vi "Error Manager Main.vi"(8 "error in (no error)":errorcluster) -> ()   [LabVIEW 2019]
uses:
  Stop Button/SubVI/Get Stop Button Status.vi
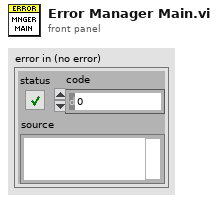
[diagram p1: front panel]
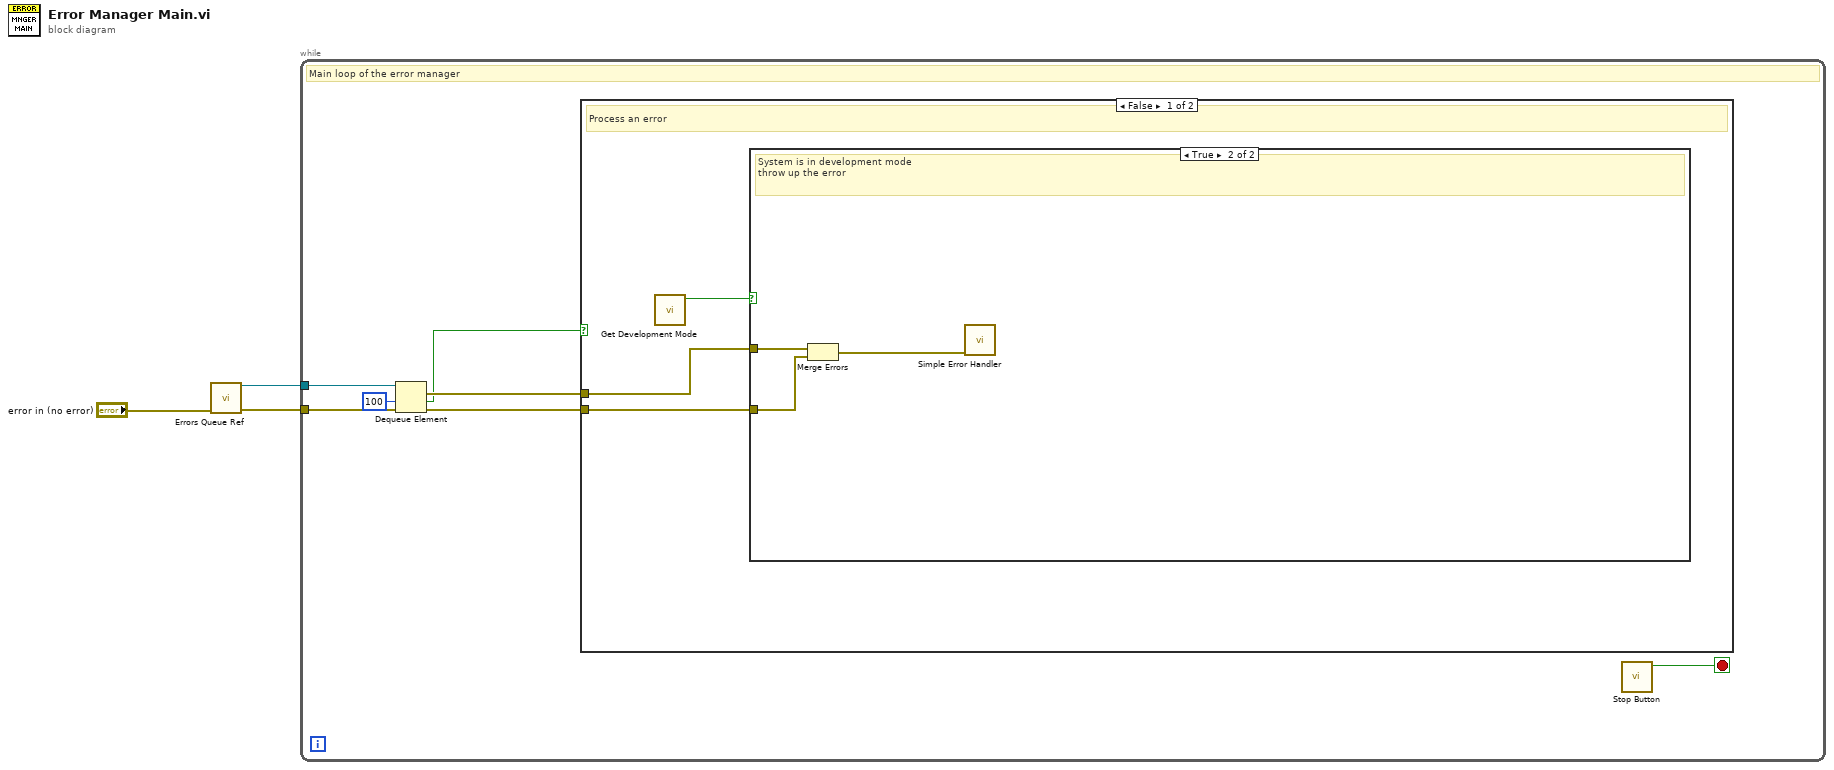
[diagram p0: block diagram]
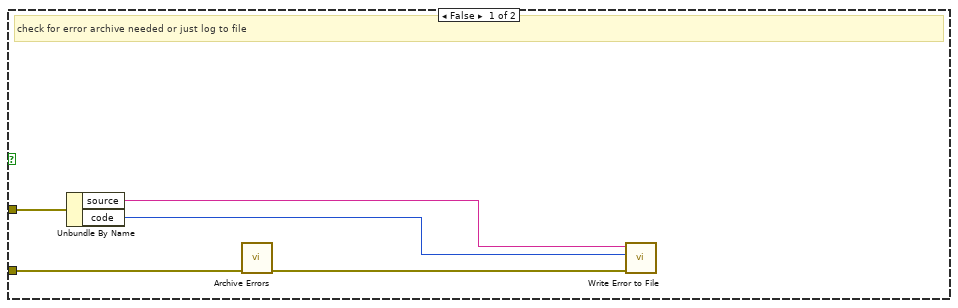
[diagram p2: hidden frame]
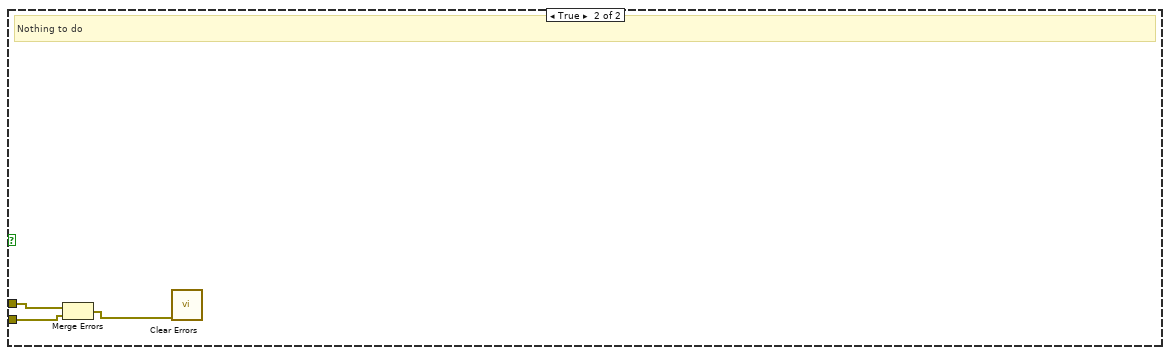
[diagram p3: hidden frame]
diagram:
  n1 = call "Errors Queue Ref.vi"("error in (no error)"="error in (no error)") -> ("error out"=w2:errorcluster, "queue out"=w3:refnum<queue>)  [unwired: 9 in]
  n2 = while {
    tunnel: w3 -> [w10]
    tunnel: w2 -> [w9]
    stop <- w7 stop-if-true
    # "Main loop of the error manager"
    n3 = Dequeue Element(queue=w10, timeout in ms (-1)=100, error in (no error)=w9) -> (element=w6:errorcluster, timed out?=w4:bool, error out=w5:errorcluster)  [unwired: 1 out]
    n4 = case shown="False" w4 {
      tunnel: w6 -> [w13 w24]
      tunnel: w5 -> [w12 w23]
      frame False {
        # "Process an error"
        n5 = call "Get Development Mode.vi"() -> ("Development"=w11:bool)  [unwired: 10 in, 1 out]
        n6 = case shown="True" w11 {
          tunnel: w13 -> [w18 w20]
          tunnel: w12 -> [w15 w21]
          frame False {
            # "check for error archive needed or just log to file"
            n7 = Unbundle By Name(w18) -> ("source"=w17:string, "code"=w16:i32)
            n8 = call "Archive Errors.vi"("Error In"=w15) -> ("error out"=w14:errorcluster)  [unwired: 10 in]
            n9 = call "Write Error to File.vi"("Error In"=w14, "Error code"=w16, "string"=w17) -> ()  [unwired: 8 in, 1 out]
          }
          frame True {
            # "System is in development mode\nthrow up the error"
            n10 = Merge Errors(w20, w21) -> (w19:errorcluster)
            n11 = call <vilib>:"Simple Error Handler.vi"("error in (no error)"=w19) -> ()  [unwired: 4 in, 5 out]
          }
        }
      }
      frame True {
        # "Nothing to do"
        n12 = Merge Errors(w24, w23) -> (w22:errorcluster)
        n13 = call <vilib>:"Clear Errors.vi"("error in (no error)"=w22) -> ()  [unwired: 5 in, 2 out]
      }
    }
    n14 = call-poly "Stop Button.vi"() -> ("Stop ButtonOut"=w7:bool)  [unwired: 10 in, 1 out]
  }
